vi "H5PTis_valid.vi"(3 "table_id":i32, 9 "error in (no error)":errorcluster) -> (0 "status":i32, 6 "error out":errorcluster)   [LabVIEW 2009]
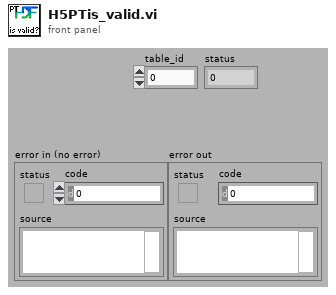
[diagram p1: front panel]
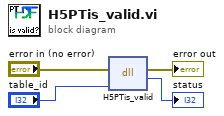
[diagram p0: block diagram]
diagram:
  n1 = dll-call lib="hdf5_hldll" fn="H5PTis_valid"(error in="error in (no error)", "table_id"="table_id") -> (error out=→"error out":errorcluster, "return type"=→"status":i32)  [unwired: 3 in, 1 out]
